vi "mpps_keithley-2400.vi"(0 "Array in":refnum<vi>, 1 "File path of JV log":path, 2 "VISA resource name":refnum<visa-resource-name>, 5 "User Name":string, 7 "Experiment Title":string, 9 "Cell details cluster":T1, 12 "Intensity (no. of suns)":string, 13 "Stabilisation time step (s)":dbl, 14 "Scan settings":T2 {"J-t settling delay (ms)" min=10.0; "J-t illumination" items=["Light only", "Dark only", "Light then dark", "Dark then light"]; "Measurement speed" items=["Fast", "Normal", "High accuracy"]; "Illumination" items=["Light only", "Dark only", "Light then dark", "Dark then light"]; "Only repeat for best pixel" items=["only for best pixel", "for best 2 pixels", "for best 3 pixels", "for best 4 pixels", "for best 5 pixels", "for best 6 pixels", "for best 7 pixels", "for all pixels"]; "No. of repeat scans" min=1.0 step=1.0; "Max power best pixel only" items=["only the best pixel", "the best 2 pixels", "the best 3 pixels", "the best 4 pixels", "the best 5 pixels", "the best 6 pixels", "the best 7 pixels", "all pixels"]; "J-t best pixel only" items=["only the best pixel", "the best 2 pixels", "the best 3 pixels", "the best 4 pixels", "the best 5 pixels", "the best 6 pixels", "the best 7 pixels", "all pixels"]; "J-t measurement speed" items=["Fast", "Normal", "High Accuracy"]; "Stabilisation mode" items=["V", "I"]; "Settling delay (ms)" min=10.0}) -> (4 "VISA Refnum out":refnum<visa-resource-name>, 6 "File path for Jt image":path, 8 "Light or dark":string, 10 "File path for Jt data":path)   [LabVIEW 2016]
uses:
  TypeDefs/scan_settings.ctl
  <instrlib>/Keithley 24XX/Keithley 24XX.lvlib
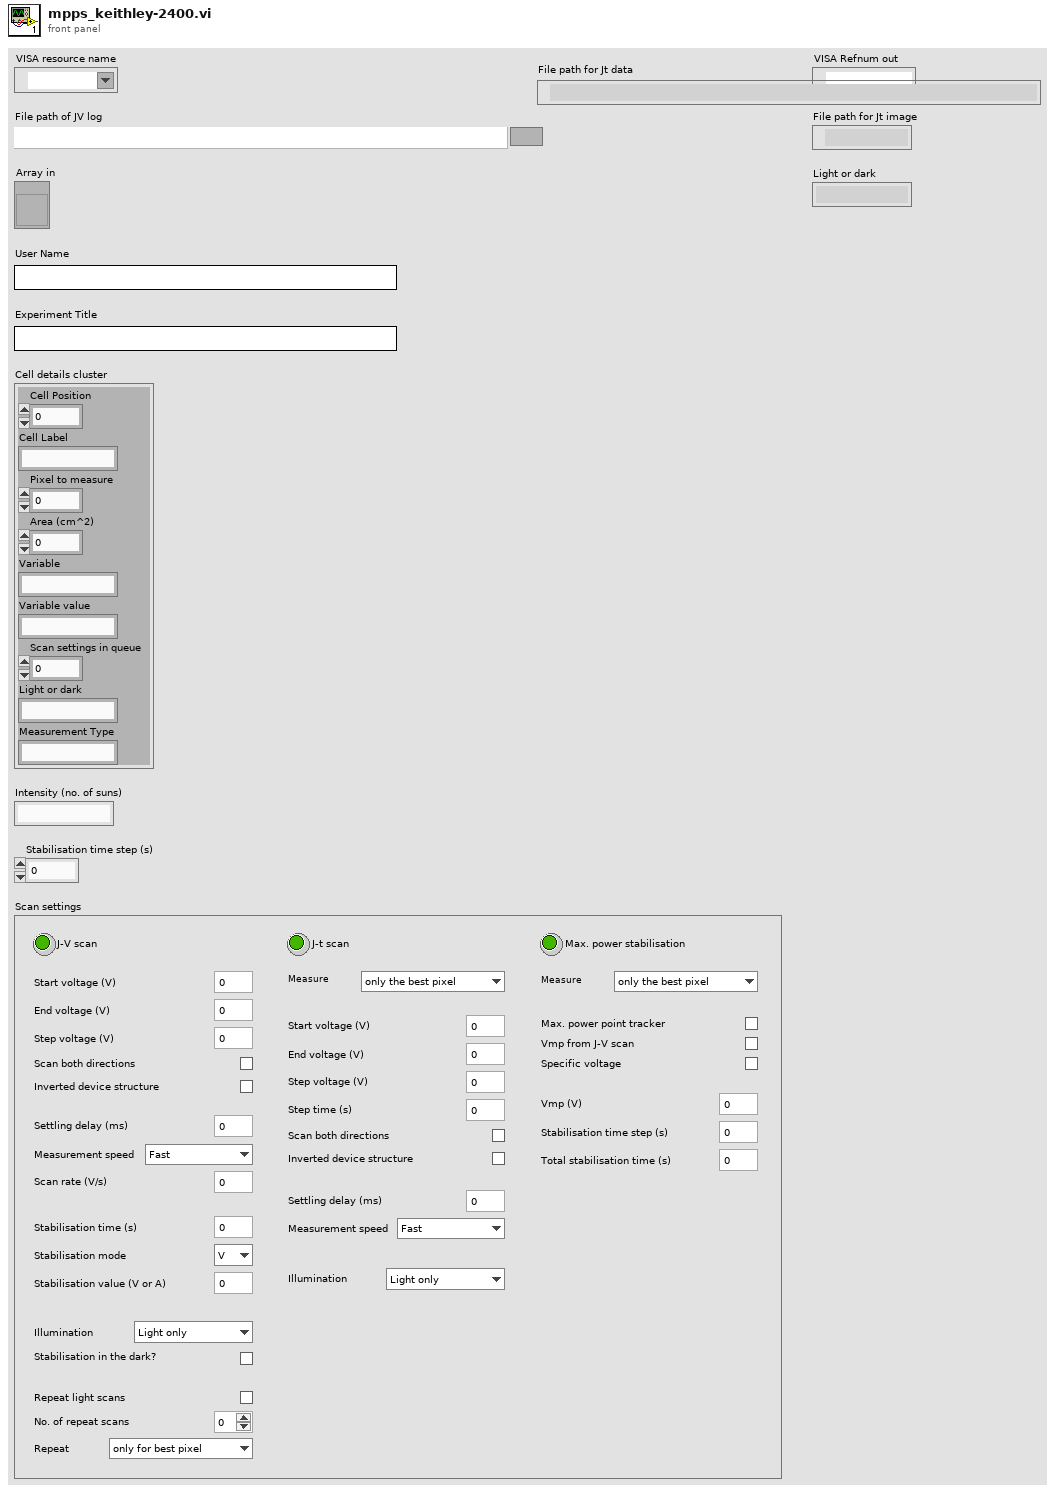
[diagram p1: front panel]
types:
  T1 = cluster{"Cell Position":i32, "Cell Label":string, "Pixel to measure":u16, "Area (cm^2)":dbl, "Variable":string, "Variable value":string, "Scan settings in queue":u16, "Light or dark":string, "Measurement Type":string}
  T2 = typedef "scan_settings.ctl" = cluster{"J-V scan":bool, "Start voltage (V)":dbl, "End voltage (V)":dbl, "Step voltage (V)":dbl, "Scan both directions":bool, "Inverted device structure":bool, "Settling delay (ms)":dbl, "Measurement speed":u8, "Scan rate (V/s)":dbl, "Stabilisation time (s)":dbl, "Stabilisation mode":u16, "Stabilisation value (V or A) ":dbl, "Illumination":u16, "Stabilisation in the dark?":bool, "Repeat light scans":bool, "No. of repeat scans":dbl, "Only repeat for best pixel":u16, "J-t scan":bool, "J-t best pixel only":u16, "J-t start voltage (V)":dbl, "J-t end voltage (V)":dbl, "J-t step voltage (V)":dbl, "Step time (s)":dbl, "J-t scan both directions":bool, "J-t inverted device structure":bool, "J-t settling delay (ms)":dbl, "J-t measurement speed":u16, "J-t illumination":u16, "Max. power stabilisation":bool, "Max power best pixel only":u16, "Max. power point tracker":bool, "Vmp from J-V scan":bool, "Max P stab. Specific voltage":bool, "Vmp (V)":dbl, "Stabilisation time step (s)":dbl, "Total stabilisation time (s)":dbl}
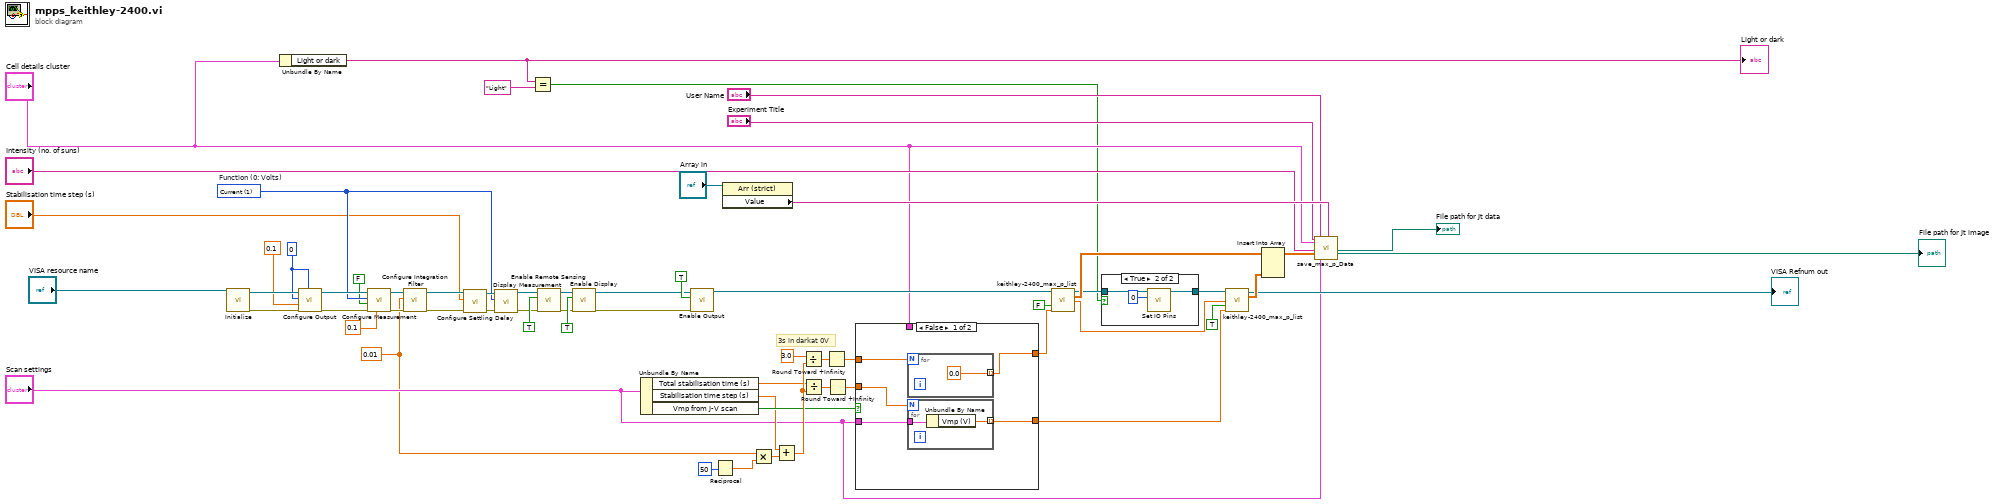
[diagram p0: block diagram]
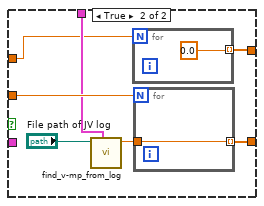
[diagram p3: hidden frame]
diagram:
  w31 = 0
  w5 = 0.01
  w23 = u16 1 items=["Volts", "Current", "Resistance"]  # Function (0: Volts)
  # "3s in darkat 0V"
  n1 = call <instrlib>:"Initialize.vi"("VISA resource name"="VISA resource name") -> ("error out"=w36:errorcluster, "VISA resource name out"=w33:refnum<visa-resource-name>)  [unwired: 4 in, 5 out]
  n2 = Unbundle By Name("Cell details cluster") -> ("Light or dark"=w13:string)
  "Light or dark" <- w13
  n3 = call <instrlib>:"Configure Output.vi"("Source Mode  (0: Voltage)"=w31, "error in (no error)"=w36, "Compliance  Level (0.1)"=0.1, "Output Level (0)"=w31, "VISA resource name"=w33) -> ("error out"=w35:errorcluster, "VISA resource name out"=w34:refnum<visa-resource-name>)  [unwired: 5 in]
  n4 = call <instrlib>:"Configure Measurement.vi"("Manual Range (1.0)"=0.1, "error in (no error)"=w35, "Enable Auto Range (T:Enable)"=FALSE, "Function (0: Volts)"=w23, "VISA resource name"=w34) -> ("error out"=w18:errorcluster, "VISA resource name out"=w19:refnum<visa-resource-name>)  [unwired: 5 in]
  n5 = call <instrlib>:"Configure Integration Filter.vi"("error in (no error)"=w18, "Measurement Speed (1 PLC)"=w5, "VISA resource name"=w19) -> ("error out"=w28:errorcluster, "VISA resource name out"=w25:refnum<visa-resource-name>)  [unwired: 7 in]
  n6 = call <instrlib>:"Configure Settling Delay.vi"("error in (no error)"=w28, "Manual Settling Delay (0 sec)"="Stabilisation time step (s)", "VISA resource name"=w25) -> ("error out"=w27:errorcluster, "VISA resource name out"=w26:refnum<visa-resource-name>)  [unwired: 7 in]
  n7 = call <instrlib>:"Display Measurement.vi"("error in (no error)"=w27, "Displayed Measurement (0: Voltage)"=w23, "VISA resource name"=w26) -> ("error out"=w16:errorcluster, "VISA resource name out"=w17:refnum<visa-resource-name>)  [unwired: 7 in]
  n8 = Equal?(x=w13, y="Light") -> (x = y?=w6:bool)
  n9 = call <instrlib>:"Enable Remote Sensing.vi"("error in (no error)"=w16, "Enable Remote Sensing (T: Enable)"=TRUE ("Enable Output (T: Enable)"), "VISA resource name"=w17) -> ("error out"=w21:errorcluster, "VISA resource name out"=w20:refnum<visa-resource-name>)  [unwired: 7 in]
  n10 = call <instrlib>:"Enable Display.vi"("error in (no error)"=w21, "Enable Display (T: Enable)"=TRUE ("Enable Output (T: Enable)"), "VISA resource name"=w20) -> ("error out"=w4:errorcluster, "VISA resource name out"=w3:refnum<visa-resource-name>)  [unwired: 7 in]
  n11 = Unbundle By Name("Scan settings") -> ("Total stabilisation time (s)"=w44:dbl, "Stabilisation time step (s)"=w43:dbl, "Vmp from J-V scan"=w47:bool)
  n12 = call <instrlib>:"Enable Output.vi"("error in (no error)"=w4, "Enable Output (T: Enable)"=TRUE ("Output (Off)"), "VISA resource name"=w3) -> ("VISA resource name out"=w55:refnum<visa-resource-name>)  [unwired: 7 in, 1 out]
  n13 = Reciprocal(x=50) -> (1/x=w40:dbl)
  n14 = property class="Arr (strict)"(reference="Array in") -> ("Value"=w63:string[])  [unwired: 1 in, 2 out]
  n15 = Multiply(x=w5, y=w40) -> (x*y=w42:dbl)
  n16 = Add(x=w43, y=w42) -> (x+y=w48:dbl)
  n17 = Divide(x=3.0, y=w48) -> (x/y=w51:dbl)
  n18 = Divide(x=w44, y=w48) -> (x/y=w50:dbl)
  n19 = Round Toward +Infinity(x=w51) -> (ceil(x): smallest int >= x=w52:dbl)
  n20 = Round Toward +Infinity(x=w50) -> (ceil(x): smallest int >= x=w45:dbl)
  n21 = case shown="False" w47 {
    tunnel: w45 -> [w68 w77]
    tunnel: "Scan settings" -> [w66 _]
    tunnel: [w67 w76] -> w46
    tunnel: "Cell details cluster" -> [_ w75]
    tunnel: w52 -> [w65 w74]
    tunnel: [w64 w73] -> w54
    frame False {
      n22 = for {
        N: w65 -> [_]
        tunnel: [0.0 ("Vmp")] -> w64 mode=indexing
      }
      n23 = for {
        N: w68 -> [_]
        tunnel: w66 -> [w71]
        tunnel: [w70] -> w67 mode=indexing
        n24 = Unbundle By Name(w71) -> ("Vmp (V)"=w70:dbl)
      }
    }
    frame True {
      n25 = call "find_v-mp_from_log.vi"("Cell details cluster in"=w75, "File path of JV log"="File path of JV log") -> ("Vmp"=w72:dbl)  [unwired: 9 in]
      n26 = for {
        N: w74 -> [_]
        tunnel: [0.0 ("Vmp")] -> w73 mode=indexing
      }
      n27 = for {
        N: w77 -> [_]
        tunnel: [w80] -> w76 mode=indexing
        tunnel: w72 -> [w80]
      }
    }
  }
  n28 = call "keithley-2400_max_p_list.vi"("VISA resource name in"=w55, "Light?"=FALSE, "Voltage List"=w54) -> ("VISA resource name out"=w58:refnum<visa-resource-name>, "Data Array"=w60:dbl[][], "timestamp"=w59:sgl)  [unwired: 9 in, 1 out]
  n29 = case shown="True" w6 {
    tunnel: w58 -> [w81 w83]
    tunnel: [w81 w82] -> w53
    frame False {
    }
    frame True {
      n30 = call <instrlib>:"Set IO Pins.vi"("Output Pattern (0)"=0, "VISA resource name"=w83) -> ("VISA resource name out"=w82:refnum<visa-resource-name>)  [unwired: 8 in, 1 out]
    }
  }
  n31 = call "keithley-2400_max_p_list.vi"("VISA resource name in"=w53, "t=0 timestamp"=w59, "Light?"=TRUE, "Voltage List"=w46) -> ("VISA resource name out"=→"VISA Refnum out":refnum<visa-resource-name>, "Data Array"=w61:dbl[][])  [unwired: 8 in, 2 out]
  n32 = Insert Into Array(array=w60, new element=w61) -> (w62:dbl[][])  [unwired: 2 in]
  n33 = call "save_max_p_Data.vi"("Experiment Indicator"="Experiment Title", "Cell details cluster"="Cell details cluster", "Intensity (no. of suns)"="Intensity (no. of suns)", "Data Array"=w62, "Username"="User Name", "Scan settings"="Scan settings", "Date array"=w63) -> ("File path for Jt data"=→"File path for Jt data":path, "File path for Jt image"=→"File path for Jt image":path)  [unwired: 9 in, 2 out]
